vi "EventLog.CreateError(single).vi"(4 "Level (Error)":T2=enum."Error", 6 "Code (-1)":i32=-1, 7 "Source (All)":T1, 8 "error in":errorcluster, 9 "arg":variant, 10 "msg":T3, 11 "create (T)":bool=TRUE) -> (0 "error out":errorcluster)   [LabVIEW 2016]
uses:
  Translator/Translator.Message.ctl
  EventLog.EventLevel.ctl
  EventLog.EventSource.ctl
  EventLog.New(single).vi
  Global/ApplicationGlobal.vi
  EventLog.Buffer.vi
  EventLog.File.ReadWrite.vi
  Tma.lib/string.llb/Join array to string.vi
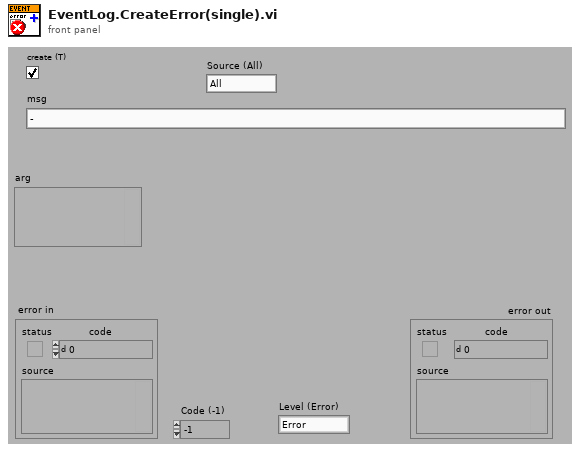
[diagram p1: front panel]
types:
  T1 = typedef "EventLog.EventSource.ctl" = enum16{"All", "Gui", "Cache", "PLC1", "PLC2", "PLC3", "DB", "DB01", "DB02", "DB03", "DB04", "DB05", "DB06", "DB07", "DB08", "DB09", "DB10", "DB11", "DB12", "DB13", "DB14", "DB15", "DB16"}
  T2 = typedef "EventLog.EventLevel.ctl" = enum8{"Debug", "Info", "Warning", "Error"}
  T3 = typedef "Translator.Message.ctl" = enum16{"-", "Event confirmed", "Log out", "Log in", "Shutdown", "Cancel", "Start", "Continue", "Stop", "On", "Off", "OK", "NOK", "NOK %s", "This", "Prev", "Home", "Work", "In progress...", "Missing", "Empty", "Hardware failure", "Initial", "Error %d >> %s", "Error %d >> %s >> %s", "Starting %s", "Quitting %s", "Configured", "Initializing", "Quitting", "Loading", "Running %s", "Stopped", "Summary", "Do you want to continue?", "Do you want to exit?", "Log out?", "System", "All", "IDLE", "Translating...%s", "Not found", "Alarm %s", "Run", "Skip", "Abort", "Repeat", "Please wait...", "Database disconnected", "Login to database successful", "Login to database failed: %d; %s", "Get process step data for %s", "Changeover off", "Changeover into %s", "Product %s | %s found in cache with status %d at previous station", "Product %s | %s found in database with status %d at previous station", "Product %s | %s not found in cache at previous station", "Product %s | %s not found in database at previous station", "Product %s | %s found in cache with status %d at this station (%d repetion)", "Product %s | %s found in database with status %d at this station (%d repetition)", "Product %s | %s not found in cache at this station", "Product %s | %s not found in database at this station", "Product %s | %s found in cache for component %s | %s", "Product %s | %s found in database for component %s | %s", "Product not found in cache for component %s | %s", "Product not found in database for component %s | %s", "Product %s | %s connected with component %s | %s (cache)", "Product %s | %s connected with component %s | %s (database)", "New data for %s | %s (cache)", "New data for %s | %s (database)", "File %s moved (cache)", "File %s deleted (cache)", "Msg %d >> %s", "PLC LifeBit Failure", "Reconnecting DB", "Reconnecting PLC", "Free disk space is below 1GB - contact technician"}
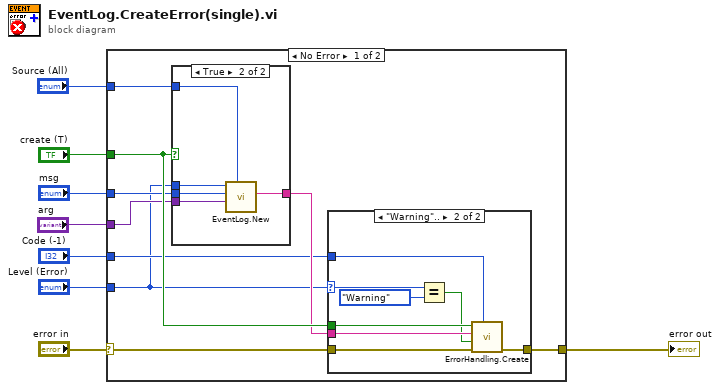
[diagram p0: block diagram]
diagram:
  n1 = case shown="No Error" "error in" {
    selector: "error in" -> [w16 w32]
    tunnel: [w15 w32] -> w8
    tunnel: "create (T)" -> [w17 _]
    tunnel: "msg" -> [w14 _]
    tunnel: "arg" -> [w13 _]
    tunnel: "Code (-1)" -> [w11 _]
    tunnel: "Level (Error)" -> [w10 _]
    tunnel: "Source (All)" -> [w9 _]
    frame No Error {
      n2 = case shown="True" w17 {
        tunnel: w14 -> [_ w31]
        tunnel: w13 -> [_ w30]
        tunnel: [_ w29] -> w12
        tunnel: w10 -> [_ w28]
        tunnel: w9 -> [_ w27]
        frame False {
        }
        frame True {
          n3 = call-poly "EventLog.New.vi"("Source (All)"=w27, "Arg"=w30, "Message (-)"=w31, "Level (Info)"=w28) -> ("Translated Msg"=w29:string)  [unwired: 6 in, 1 out]
        }
      }
      n4 = case shown="\"Warning\".." w10 {
        selector: w10 -> [_ w21]
        tunnel: w17 -> [_ w26]
        tunnel: w16 -> [w18 w25]
        tunnel: [w18 w24] -> w15
        tunnel: w12 -> [_ w23]
        tunnel: w11 -> [_ w22]
        frame Default {
        }
        frame "Warning".. {
          n5 = Equal?(x=w21, y=EventLog.EventLevel."Warning") -> (x = y?=w19:bool)
          n6 = call "ErrorHandling.Create.vi"("error code (5000)"=w22, "error in"=w25, "warning only (F)"=w19, "explanation"=w23, "create (T)"=w26) -> ("error out"=w24:errorcluster)  [unwired: 6 in]
        }
      }
    }
    frame Error {
    }
  }
  "error out" <- w8
